vi "MatrixSwitch.vi"(8 "error in (no error)":errorcluster, 10 "Action":T1(ring), 11 "Switching in":refnum<class "Switching.lvclass">) -> (0 "error out":errorcluster, 2 "Continue?":bool, 3 "Switching out":refnum<class "Switching.lvclass">)   [LabVIEW 2019, in "Switching.lvclass"]
uses:
  Switching.lvclass
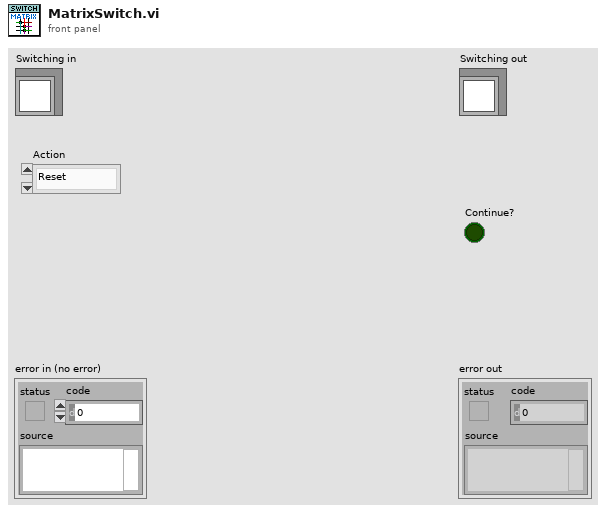
[diagram p1: front panel]
types:
  T1 = enum16{"Reset", "Ground", "Striptest Bias", "Striptest SMU", "Striptest LCR", "IV", "CV", "Interstrip Cap", "Interstrip Res", "PTP", "Implant Resistance", "Metal Resistance", "Coupling Capacitance"}
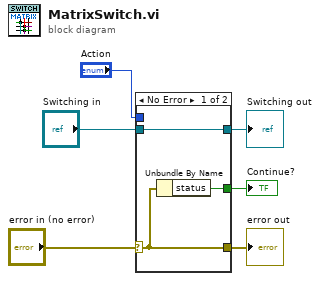
[diagram p0: block diagram]
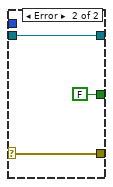
[diagram p2: hidden frame]
diagram:
  n1 = case shown="No Error" "error in (no error)" {
    selector: "error in (no error)" -> [w8 w12]
    tunnel: [w8 w12] -> w6
    tunnel: [w7 w11] -> w5
    tunnel: "Switching in" -> [w7 w11]
    tunnel: [w9 FALSE] -> w4
    tunnel: "Action" -> [_ _]
    frame No Error {
      n2 = Unbundle By Name(w8) -> ("status"=w9:bool)
    }
    frame Error {
    }
  }
  "error out" <- w6
  "Switching out" <- w5
  "Continue?" <- w4
